vi "PathDrawerMain.vi"() -> ()   [LabVIEW 2017]
panel:
  in  "Load From File":bool
  in  "Starting Position Preset":enum16{"1", "2", "3", "4", "No Preset"}(ring)=enum."3"
  in  "PointSpacing":dbl=12.0 min=1.0 format="%#_13g"
  in  "CenterOfRotYOffset":dbl=20.0
  in  "PathMode":enum16{"Left", "Right", "Center"}(ring)=enum."Center"
  in  "RobotWidth":dbl=30.0
  in  "RobotLength":dbl=40.0
  in  "Roundedness":dbl(slide)=0.7875252525252525 scale=0.6..0.995
  in  "Export To File":bool
  in  "Points":cluster{dbl, dbl}[](array[cluster])=[{46.0, 206.0}, {72.0, 199.0}, {97.0, 267.0}, {149.0, 262.0}]
  out "Path Drawer":T1(plugin-control)
  # "MORE INSTRUCTIONS"
  # "Use a preset if your path starts\nat one of the presets. \n\n(Click it multiple times please)"
  # "Includes bumpers"
  # "Relative to outside face of\nback bumber of robot"
  # "INSTRUCTIONS"
  # "The red line is the path that the robot recieves. Everything else is to help create that path\n\nUse the multi-line tool to draw a path. Double click to stop drawing.\nHover over a node and press backspace to remove it.\nPress I to insert a new node (at the end of the path only, for now)\n\nUse the contols to input robot width, height, and center of rotation offset,\nHow far apart the points in the \"real world units\" path are,\nWhether the robot travels on the left or right of your green lines, and\nthe roundedness of the path. (Note: point spacing affects roundedness)\n\nYou can manually edit the green node's location in the path with the Points array,\nor drag the nodes on the image\n\nPress Export To File and enter the file name (no extension) to save the path to a file in the\nThisVIsDirectory\\Paths\\ folder\n\nIf you acidentally clear your path press Z quickly to get it back"
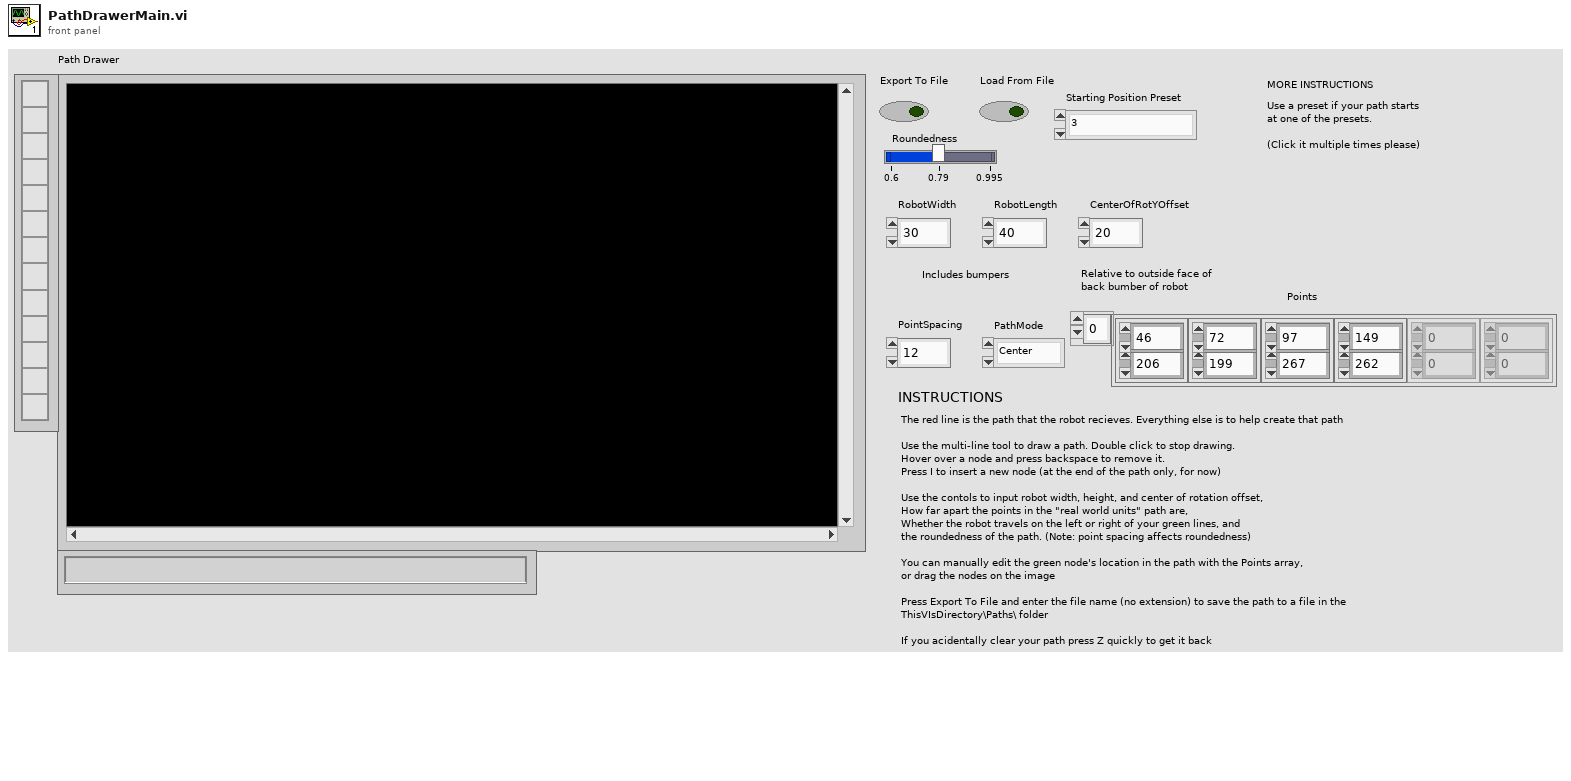
[diagram p1: front panel]
types:
  T1 = typedef "IMAQ Image.ctl" = refnum<image>
  T2 = typedef "Image Type" = u32
  T3 = cluster{"Path (px)":cluster{i32, i32}[], "RobotLength":dbl, "RobotWidth":dbl, "CenterOfRotYOffset":dbl, "Roundedness":dbl, "PointSpacing":dbl}
  T4 = cluster{"PathData":cluster{"Path":cluster{dbl, dbl}[]}}
  T5 = cluster{"Global Rectangle":i32[], "Contours":cluster{"Contour Type":u32, "ROI Type":u32, "Points":i32[]}[]}
  T6 = cluster{"Contour Type":u32, "ROI Type":u32, "Points":i32[]}[]
  T7 = cluster{"Contour Type":u32, "ROI Type":u32, "Points":i32[]}
  T8 = cluster{"PathData":cluster{"Path":cluster{dbl, dbl}[]}, "MetaData":cluster{"Path (px)":cluster{i32, i32}[]}}
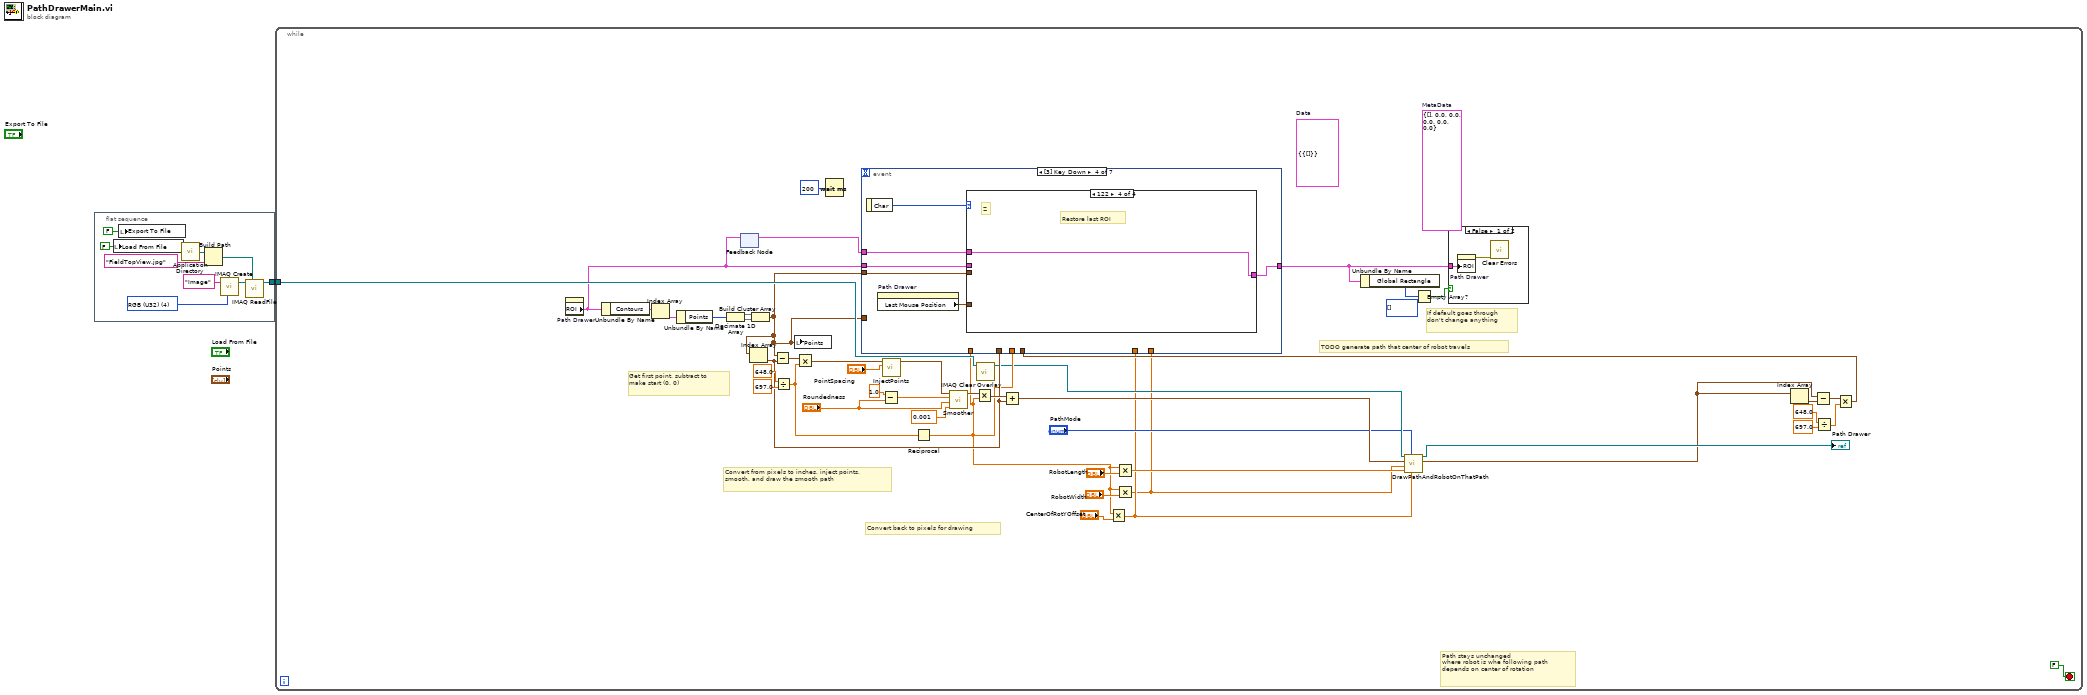
[diagram p0: block diagram]
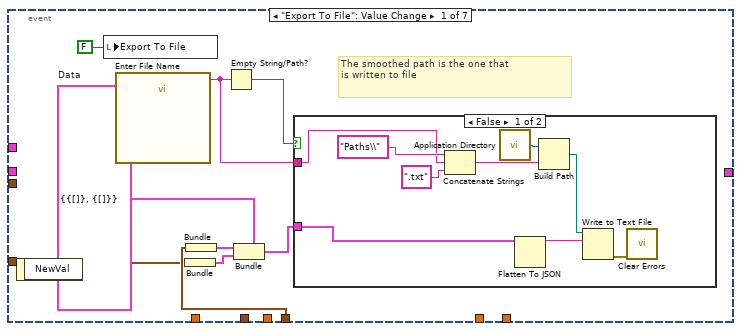
[diagram p3: hidden frame]
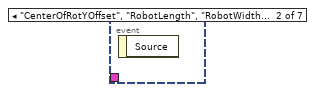
[diagram p5: hidden frame]
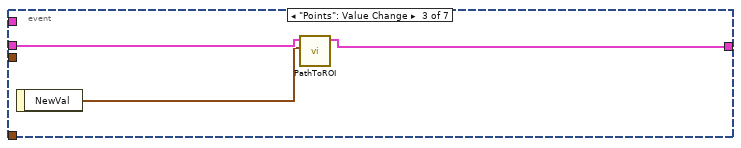
[diagram p6: hidden frame]
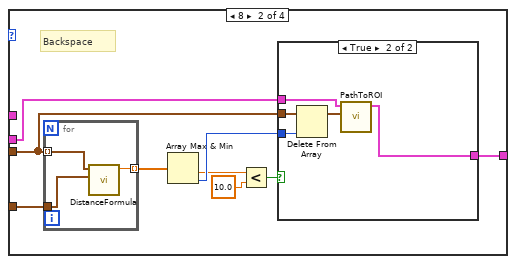
[diagram p8: hidden frame]
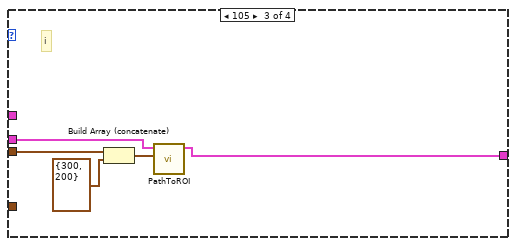
[diagram p10: hidden frame]
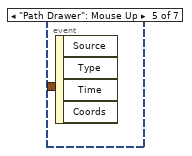
[diagram p11: hidden frame]
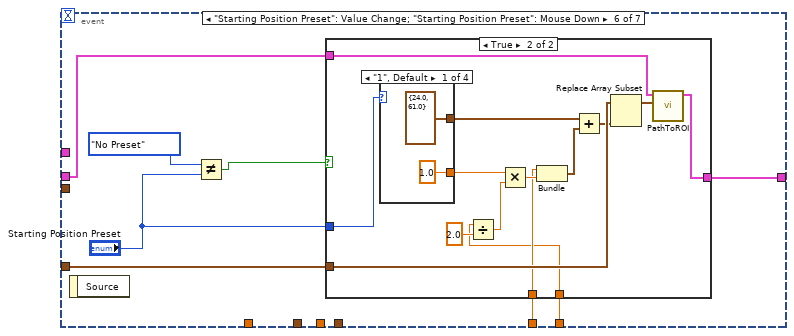
[diagram p12: hidden frame]
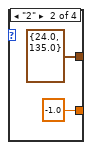
[diagram p14: hidden frame]
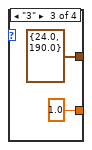
[diagram p15: hidden frame]
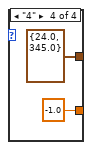
[diagram p16: hidden frame]
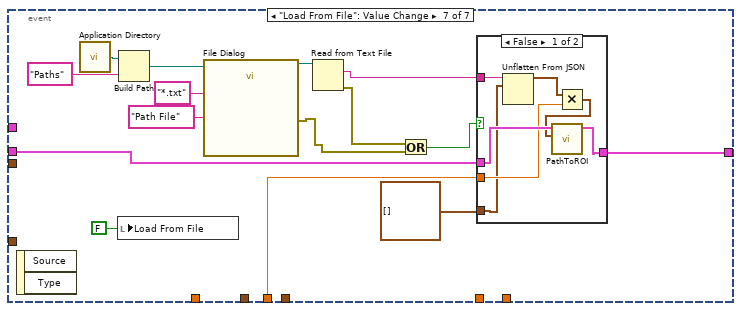
[diagram p17: hidden frame]
diagram:
  n1 = flat-sequence {
    tunnel: [w4] -> w1
    frame #0 {
      w6 = T2 4 items=["Grayscale (U8)", "Grayscale (I16)", "Grayscale (SGL)", "Complex (CSG)", "RGB (U32)", "HSL (U32)", "RGB (U64)", "Grayscale (U16)"] ("Image Type")
      n2 = local write "Load From File"(FALSE ("Export To File")) -> ()
      n3 = local write "Export To File"(FALSE ("Export To File")) -> ()
      n4 = call <vilib>:"Application Directory.vi"() -> ("Application Directory"=w10:path)
      n5 = Build Path(base path=w10, name or relative path="FieldTopView.jpg") -> (appended path=w8:path)
      n6 = call "IMAQ Create"("Image Name"="Image", "Image Type"=w6) -> ("New Image"=w5:T1)  [unwired: 3 in, 1 out]
      n7 = call "IMAQ ReadFile"("File Path"=w8, "Image"=w5) -> ("Image Out"=w4:T1)  [unwired: 5 in, 4 out]
    }
  }
  n8 = while {
    tunnel: w1 -> [w48]
    stop <- FALSE stop-if-true
    (unwired) T3 {"Path (px)"=[], "RobotLength"=0.0, "RobotWidth"=0.0, "CenterOfRotYOffset"=0.0, "Roundedness"=0.0, "PointSpacing"=0.0}  # MetaData
    (unwired) T4 {"PathData"={"Path"=[]}}  # Data
    (unwired) i32[] [] ("Global Rectangle")
    # "Path stays unchanged\nwhere robot is whe following path\ndepends on center of rotation"
    # "Convert back to pixels for drawing"
    # "TODO generate path that center of robot travels"
    # "If default goes through\ndon't change anything"
    # "Convert from pixels to inches, inject points,\nsmooth, and draw the smooth path"
    # "Get first point, subtract to\nmake start (0, 0)"
    n9 = property on="Path Drawer" class="ImageControl"() -> ("ROI"=w23:T5)  [unwired: 2 in, 2 out]
    n10 = Unbundle By Name(w23) -> ("Contours"=w55:T6)
    n11 = Index Array(array=w55) -> (element=w50:T7)  [unwired: 1 in]
    n12 = Unbundle By Name(w50) -> ("Points"=w43:i32[])
    n13 = Decimate 1D Array(w43) -> (w54:i32[], w53:i32[])
    n14 = feedback-in #1(w23) -> ()
    n15 = feedback #1() -> (w21:T5)  [unwired: 1 in]
    n16 = Build Cluster Array(w54, w53) -> (w22:cluster{i32, i32}[])
    n17 = Index Array(array=w22) -> (element=w25:cluster{i32, i32})  [unwired: 1 in]
    n18 = Subtract(x=w22, y=w25) -> (x-y=w44:cluster{i32, i32}[])
    n19 = Divide(x=648.0, y=697.0) -> (x/y=w49:dbl)
    n20 = local write "Points"(w22) -> ()
    n21 = Multiply(x=w44, y=w49) -> (x*y=w26:cluster{dbl, dbl}[])
    n22 = Wait (ms)(milliseconds to wait=u32 200) -> ()  [unwired: 1 out]
    n23 = call "InjectPoints.vi"("Distance"="PointSpacing", "Path"=w26) -> ("Path out"=w46:cluster{dbl, dbl}[])  [unwired: 9 in]
    n24 = Subtract(x=1.0, y="Roundedness") -> (x-y=w41:dbl)
    n25 = Reciprocal(x=w49) -> (1/x=w19:dbl)
    n26 = call "Smoother.vi"("tolerance"=0.001, "B"="Roundedness", "A"=w41, "Path"=w46) -> ("SmoothPath"=w36:cluster{dbl, dbl}[])  [unwired: 7 in]
    n27 = Multiply(x=w36, y=w19) -> (x*y=w45:cluster{dbl, dbl}[])
    n28 = call "IMAQ Clear Overlay"("Image"=w48) -> ("Image Out"=w16:T1)  [unwired: 9 in, 1 out]
    n29 = Add(x=w45, y=w25) -> (x+y=w15:cluster{dbl, dbl}[])
    n30 = Multiply(x=w19, y="CenterOfRotYOffset") -> (x*y=w12:dbl)
    n31 = Multiply(x=w19, y="RobotLength") -> (x*y=w14:dbl)
    n32 = Multiply(x=w19, y="RobotWidth") -> (x*y=w11:dbl)
    n33 = call "DrawPathAndRobotOnThatPath.vi"("CenterOfRotYOffset (px)"=w12, "PathMode"="PathMode", "RobotLength (px)"=w14, "RobotWidth (px)"=w11, "Path (px)"=w15, "Image In"=w16) -> ("NewPath (px)"=w17:cluster{dbl, dbl}[], "Image Out"=→"Path Drawer":T1)  [unwired: 4 in]
    n34 = Index Array(array=w17) -> (element=w28:cluster{dbl, dbl})  [unwired: 1 in]
    n35 = Subtract(x=w17, y=w28) -> (x-y=w29:cluster{dbl, dbl}[])
    n36 = Divide(x=648.0, y=697.0) -> (x/y=w30:dbl)
    n37 = Multiply(x=w29, y=w30) -> (x*y=w27:cluster{dbl, dbl}[])
    n38 = event shown="[3] Key Down" {
      selector: _ -> [_ _ _ _ _ _ _]
      dyn-events: _ -> [_ _ _ _ _ _ _]
      timeout: _ -> [_ _ _ _ _ _ _]
      tunnel: w23 -> [_ _ w79 w85 _ w117 w150]
      tunnel: w22 -> [_ _ _ w84 _ _ _]
      tunnel: [_ _ w78 w81 _ w118 w151] -> w24
      tunnel: w27 -> [w61 _ _ _ _ _ _]
      tunnel: w25 -> [_ _ _ _ _ _ _]
      tunnel: w21 -> [_ _ _ w80 _ _ _]
      tunnel: w22 -> [w59 _ _ _ _ w116 _]
      tunnel: w19 -> [_ _ _ _ _ _ _]
      tunnel: w19 -> [_ _ _ _ _ _ w144]
      tunnel: w12 -> [_ _ _ _ _ w112 _]
      tunnel: w11 -> [_ _ _ _ _ w111 _]
      event "Export To File": Value Change {
        w64 = T8 {"PathData"={"Path"=[]}, "MetaData"={"Path (px)"=[]}}  # Data
        # "The smoothed path is the one that\nis written to file"
        n39 = event-data() -> ()  [unwired: 1 in, 1 out]
        n40 = local write "Export To File"(FALSE ("Export To File")) -> ()
        n41 = call "Enter File Name"() -> ("File Name"=w65:string)  [unwired: 17 in, 2 out]
        n42 = Bundle(w59) -> (w60:cluster{cluster{i32, i32}[]})  [unwired: 1 in]
        n43 = Bundle(w61) -> (w62:cluster{cluster{dbl, dbl}[]})  [unwired: 1 in]
        n44 = Empty String/Path?(string/path=w65) -> (empty?=w66:bool)
        n45 = Bundle(cluster=w64, "PathData"=w62, "MetaData"=w60) -> (w63:T8)
        n46 = case shown="False" w66 {
          tunnel: w63 -> [w68 _]
          tunnel: w65 -> [w70 _]
          frame False {
            n47 = Concatenate Strings("Paths\\" ("name or relative path"), w70, ".txt" ("string")) -> (w76:string)
            n48 = call <vilib>:"Application Directory.vi"() -> ("Application Directory"=w75:path)
            n49 = Flatten To JSON(anything=w68) -> (JSON string=w73:string)  [unwired: 2 in, 1 out]
            n50 = Build Path(base path=w75, name or relative path=w76) -> (appended path=w71:path)
            n51 = Write to Text File(file (use dialog)=w71, text=w73) -> (error out=w72:errorcluster)  [unwired: 2 in, 2 out]
            n52 = call <vilib>:"Clear Errors.vi"("error in (no error)"=w72) -> ()  [unwired: 5 in, 2 out]
          }
          frame True {
          }
        }
      }
      event "CenterOfRotYOffset", "RobotLength", "RobotWidth", "PathMode", "PointSpacing", "Roundedness": Value Change {
        n53 = event-data() -> ()  [unwired: 1 in, 1 out]
      }
      event "Points": Value Change {
        n54 = event-data() -> ("NewVal"=w77:cluster{dbl, dbl}[])  [unwired: 1 in]
        n55 = call "PathToROI.vi"("Path In"=w77, "ROI In"=w79) -> ("ROI Out"=w78:T5)  [unwired: 9 in]
      }
      event Key Down {
        n56 = event-data() -> ("Char"=w83:i16)  [unwired: 1 in]
        n57 = property on="Path Drawer" class="ImageControl"() -> ("Last Mouse Position"=w82:cluster{"X":i32, "Y":i32})  [unwired: 2 in, 2 out]
        n58 = case shown="122" w83 {
          tunnel: w85 -> [w86 w95 w107 _]
          tunnel: w84 -> [_ w94 w109 _]
          tunnel: w82 -> [_ w88 _ _]
          tunnel: [w86 w87 w105 w110] -> w81
          tunnel: w80 -> [_ _ _ w110]
          frame 0, Default {
          }
          frame 8 {
            # "Backspace"
            n59 = for {
              tunnel: w94 -> [w104] mode=indexing
              tunnel: [w103] -> w93 mode=indexing
              tunnel: w88 -> [w102]
              n60 = call "DistanceFormula.vi"("Point 2"=w102, "Point 1"=w104) -> ("Distance"=w103:dbl)  [unwired: 9 in]
            }
            n61 = Array Max & Min(array=w93) -> (min value=w91:dbl, min index (indices)=w92:i32)  [unwired: 2 out]
            n62 = Less?(x=w91, y=10.0) -> (x < y?=w89:bool)
            n63 = case shown="True" w89 {
              tunnel: w92 -> [_ w101]
              tunnel: w94 -> [_ w100]
              tunnel: w95 -> [w96 w98]
              tunnel: [w96 w97] -> w87
              frame False {
              }
              frame True {
                n64 = Delete From Array(array=w100, index=w101) -> (array with subset deleted=w99:cluster{i32, i32}[])  [unwired: 1 in, 1 out]
                n65 = call "PathToROI.vi"("Path In"=w99, "ROI In"=w98) -> ("ROI Out"=w97:T5)  [unwired: 9 in]
              }
            }
          }
          frame 105 {
            # "i"
            n66 = Build Array (concatenate)(w109, cluster{i32, i32} {300, 200}) -> (w108:cluster{i32, i32}[])
            n67 = call "PathToROI.vi"("Path In"=w108, "ROI In"=w107) -> ("ROI Out"=w105:T5)  [unwired: 9 in]
          }
          frame 122 {
            # "Restore last ROI"
            # "Z"
          }
        }
      }
      event "Path Drawer": Mouse Up {
        n68 = event-data() -> ()  [unwired: 1 in, 4 out]
      }
      event "Starting Position Preset": Value Change; "Starting Position Preset": Mouse Down {
        n69 = event-data() -> ()  [unwired: 1 in, 1 out]
        n70 = Not Equal?(x=enum16{"1", "2", "3", "4", "No Preset"}."No Preset" ("y"), y="Starting Position Preset") -> (x != y?=w114:bool)
        n71 = case shown="True" w114 {
          tunnel: [_ w131] -> w118
          tunnel: w117 -> [_ w130]
          tunnel: w116 -> [_ w128]
          tunnel: "Starting Position Preset" -> [_ w122]
          tunnel: w112 -> [_ w120]
          tunnel: w111 -> [_ w119]
          frame False {
          }
          frame True {
            n72 = case shown="\"1\", Default" w122 {
              tunnel: [cluster{dbl, dbl} {24.0, 61.0} cluster{dbl, dbl} {24.0, 135.0} cluster{dbl, dbl} {24.0, 190.0} cluster{dbl, dbl} {24.0, 345.0}] -> w132
              tunnel: [1.0 -1.0 1.0 -1.0] -> w123
              frame "1", Default {
              }
              frame "2" {
              }
              frame "3" {
              }
              frame "4" {
              }
            }
            n73 = Divide(x=w119, y=2.0) -> (x/y=w125:dbl)
            n74 = Multiply(x=w123, y=w125) -> (x*y=w124:dbl)
            n75 = Bundle(w120, w124) -> (w121:cluster{dbl, dbl})  [unwired: 1 in]
            n76 = Add(x=w132, y=w121) -> (x+y=w127:cluster{dbl, dbl})
            n77 = Replace Array Subset(array=w128, new element=w127) -> (w129:cluster{i32, i32}[])  [unwired: 1 in]
            n78 = call "PathToROI.vi"("Path In"=w129, "ROI In"=w130) -> ("ROI Out"=w131:T5)  [unwired: 9 in]
          }
        }
      }
      event "Load From File": Value Change {
        n79 = event-data() -> ()  [unwired: 1 in, 2 out]
        n80 = call <vilib>:"Application Directory.vi"() -> ("Application Directory"=w155:path)
        n81 = local write "Load From File"(FALSE ("Export To File")) -> ()
        n82 = Build Path(base path=w155, name or relative path="Paths") -> (appended path=w153:path)
        n83 = call "File Dialog"("start path"=w153, "pattern (all files)"="*.txt", "pattern label"="Path File") -> ("selected path"=w149:path, "error out"=w147:errorcluster)  [unwired: 9 in, 2 out]
        n84 = Read from Text File(file (use dialog)=w149) -> (text=w143:string, error out=w148:errorcluster)  [unwired: 3 in, 2 out]
        n85 = Or(x=w148, y=w147) -> (x .or. y?=w146:bool)
        n86 = case shown="False" w146 {
          tunnel: [w162 _] -> w151
          tunnel: w150 -> [w161 _]
          tunnel: w144 -> [w159 _]
          tunnel: w143 -> [w158 _]
          tunnel: cluster{i32, i32}[] [] ("array of clusters") -> [w157 _]
          frame False {
            n87 = Unflatten From JSON(JSON string=w158, type and defaults=w157) -> (value=w160:cluster{i32, i32}[])  [unwired: 5 in, 1 out]
            n88 = Multiply(x=w160, y=w159) -> (x*y=w156:cluster{dbl, dbl}[])
            n89 = call "PathToROI.vi"("Path In"=w156, "ROI In"=w161) -> ("ROI Out"=w162:T5)  [unwired: 9 in]
          }
          frame True {
          }
        }
      }
    }
    n90 = Unbundle By Name(w24) -> ("Global Rectangle"=w38:i32[])
    n91 = Empty Array?(array=w38) -> (empty?=w37:bool)
    n92 = case shown="False" w37 {
      tunnel: w24 -> [w57 _]
      frame False {
        n93 = property on="Path Drawer" class="ImageControl"("ROI"=w57) -> (error out=w58:errorcluster)  [unwired: 2 in, 1 out]
        n94 = call <vilib>:"Clear Errors.vi"("error in (no error)"=w58) -> ()  [unwired: 5 in, 2 out]
      }
      frame True {
      }
    }
  }
